vi "Write Subscriber.vi"(8 "error in (no error)":errorcluster, 10 "Subscriber.lvclass":refnum<class "Subscriber.lvclass">, 11 "Device Connector MSG in":refnum<class "Device Connector MSG.lvclass">) -> (0 "error out":errorcluster, 3 "Device Connector MSG out":refnum<class "Device Connector MSG.lvclass">)   [LabVIEW 2019, in "Device Connector MSG.lvclass"]
uses:
  Device Connector MSG.lvclass
  Ancestor Class/Subscriber/Subscriber.lvclass
  Device Connector MSG.lvclass/Device Connector MSG.ctl
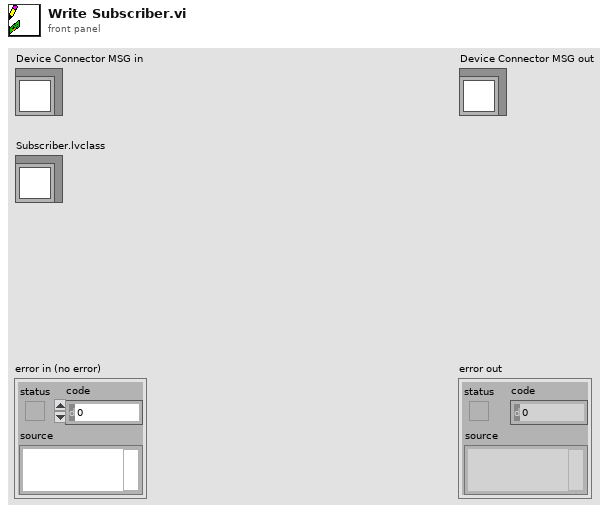
[diagram p1: front panel]
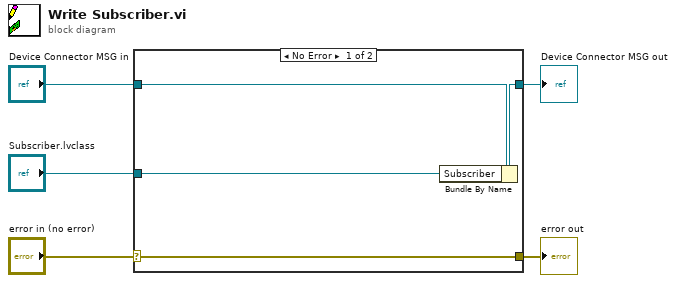
[diagram p0: block diagram]
diagram:
  n1 = case shown="No Error" "error in (no error)" {
    selector: "error in (no error)" -> [w9 w10]
    tunnel: [w9 w10] -> w4
    tunnel: [w7 w11] -> w2
    tunnel: "Device Connector MSG in" -> [w8 w11]
    tunnel: "Subscriber.lvclass" -> [w6 _]
    frame No Error {
      n2 = Bundle By Name(cluster=w8, "Subscriber"=w6) -> (w7:refnum<class "Device Connector MSG.lvclass">)
    }
    frame Error {
    }
  }
  "error out" <- w4
  "Device Connector MSG out" <- w2
